vi "Write Speaker State CMD.vi"(8 "error in (no error)":errorcluster, 10 "PAS Library.lvlib:Change Speaker State CMD":refnum<class "Change Speaker State CMD.lvclass">, 11 "PAS in":refnum<class "PAS.lvclass">) -> (0 "error out":errorcluster, 3 "PAS out":refnum<class "PAS.lvclass">)   [LabVIEW 2016, in "PAS Library.lvlib" / "PAS.lvclass"]
uses:
  PAS.lvclass
  Commands/Change Speaker State CMD/Change Speaker State CMD.lvclass
  PAS.lvclass/PAS.ctl
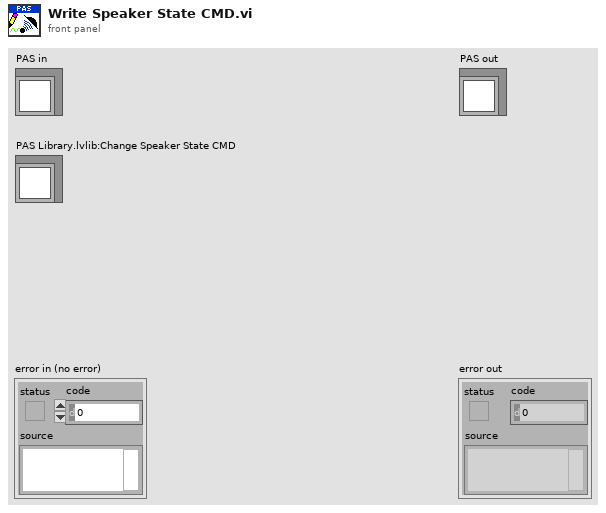
[diagram p1: front panel]
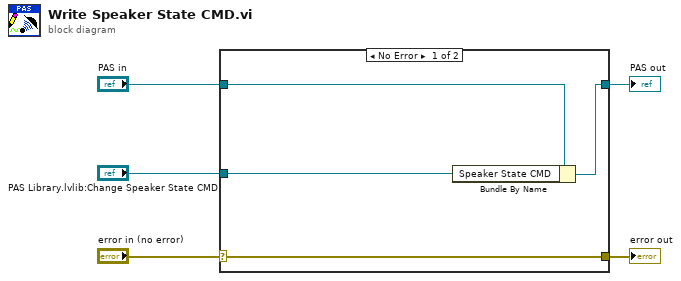
[diagram p0: block diagram]
diagram:
  n1 = case shown="No Error" "error in (no error)" {
    selector: "error in (no error)" -> [w9 w10]
    tunnel: [w9 w10] -> w4
    tunnel: [w7 w11] -> w2
    tunnel: "PAS in" -> [w8 w11]
    tunnel: "PAS Library.lvlib:Change Speaker State CMD" -> [w6 _]
    frame No Error {
      n2 = Bundle By Name(cluster=w8, "Speaker State CMD"=w6) -> (w7:refnum<class "PAS.lvclass">)
    }
    frame Error {
    }
  }
  "error out" <- w4
  "PAS out" <- w2
